vi "Tarea 2.vi"() -> ()   [LabVIEW 2019]
uses:
  Student Material/Student Material/Module 1/Exercise 2/CLD 2 Time Mode.ctl
panel:
  in  "Auto Reset (F)":bool
  in  "Time Target (s)":dbl
  in  "Timer  Mode":T1
  out "Elapsed Time (s)":dbl format="%#.3g"
  out "Time Has Elapsed":bool
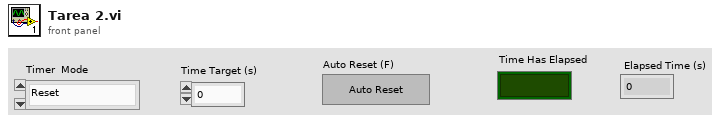
[diagram p1: front panel]
types:
  T1 = typedef "CLD 2 Time Mode.ctl" = enum16{"Reset", "Read Status", "Set Auto Reset"}
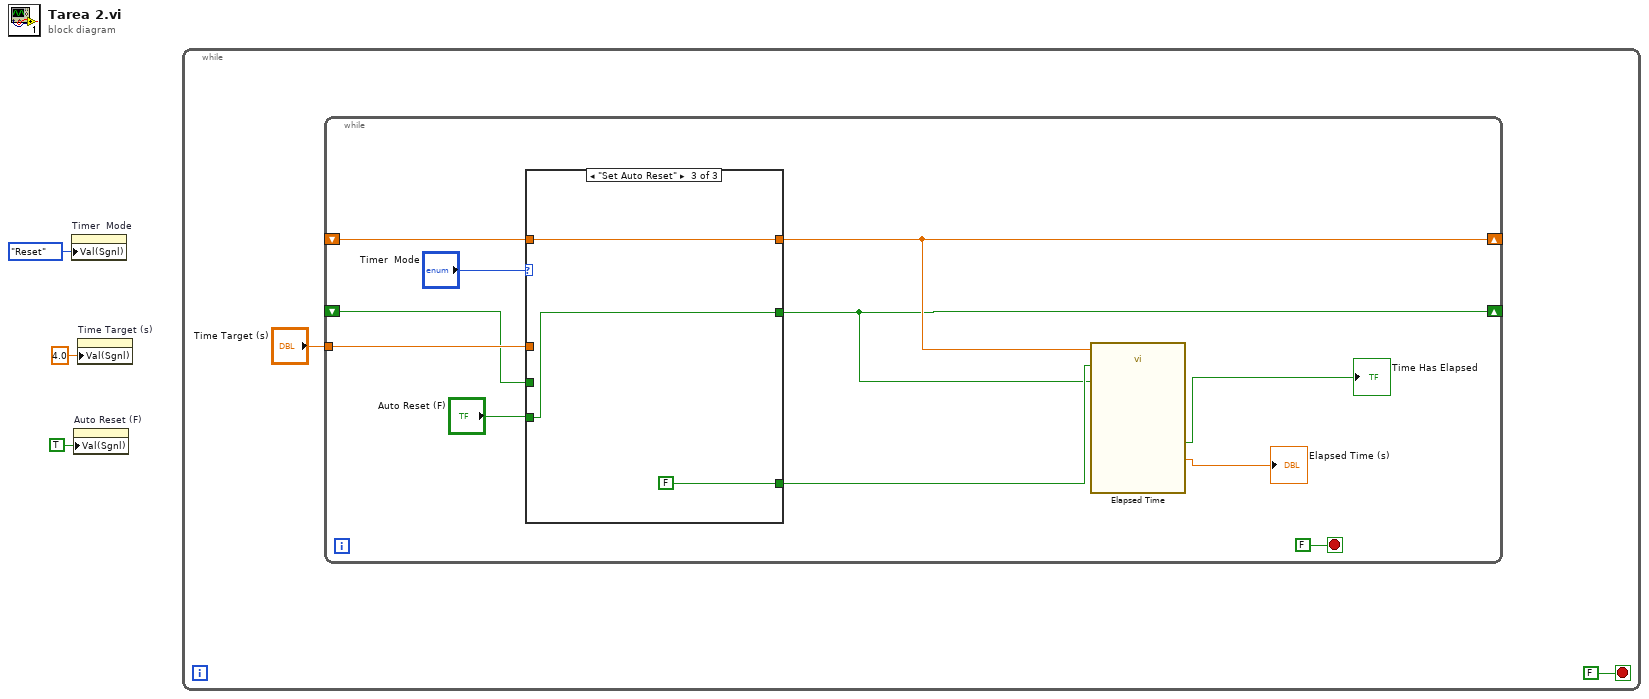
[diagram p0: block diagram]
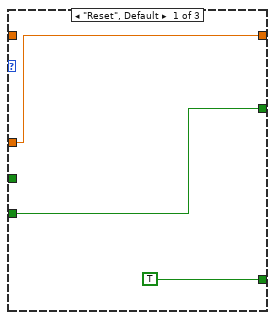
[diagram p2: hidden frame]
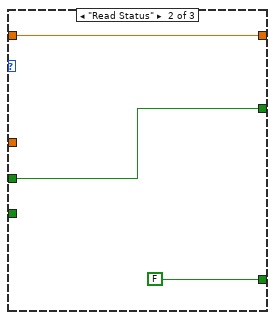
[diagram p3: hidden frame]
diagram:
  n1 = property on="Timer  Mode" class="Enum (strict)"("Val(Sgnl)"=CLD_2_Time_Mode."Reset" ("Value (Signaling)")) -> ()  [unwired: 2 in, 2 out]
  n2 = property on="Auto Reset (F)" class="Bool (strict)"("Val(Sgnl)"=TRUE ("Value (Signaling)")) -> ()  [unwired: 2 in, 2 out]
  n3 = property on="Time Target (s)" class="DigNum (strict)"("Val(Sgnl)"=4.0 ("Value (Signaling)")) -> ()  [unwired: 2 in, 2 out]
  n4 = while {
    stop <- FALSE stop-if-true
    n5 = while {
      shift-right: [w11] -> _
      shift-left: _ -> [w16]
      shift-right: [w10] -> _
      shift-left: _ -> [w14]
      tunnel: "Time Target (s)" -> [w15]
      stop <- FALSE stop-if-true
      n6 = case shown="\"Set Auto Reset\"" "Timer  Mode" {
        tunnel: w16 -> [_ w22 w25]
        tunnel: [w19 w22 w25] -> w11
        tunnel: w15 -> [w19 _ _]
        tunnel: w14 -> [_ w20 _]
        tunnel: [w18 w20 w24] -> w10
        tunnel: "Auto Reset (F)" -> [w18 _ w24]
        tunnel: [TRUE FALSE FALSE] -> w12
        frame "Reset", Default {
        }
        frame "Read Status" {
        }
        frame "Set Auto Reset" {
        }
      }
      n7 = call "Elapsed Time"("Time Target (s)"=w11, "Reset"=w12, "Auto Reset"=w10) -> ("Elapsed Time (s)"=→"Elapsed Time (s)":dbl, "Time has Elapsed"=→"Time Has Elapsed":bool)  [unwired: 9 in, 6 out]
    }
  }
